vi "Motion Magic.vi"(0 "In":dbl(knob) scale=-360.0..360.0, 1 "Cluster":T1={"kp"=0.28, "ki"=0.0, "kd"=0.02, "kv"=0.104, "ka"=0.0}, 2 "Target":dbl, 3 "Max V":dbl format="%#_13g", 4 "Velocity":dbl format="%#_13g", 5 "Max A":dbl format="%#_13g", 6 "Reset":bool) -> (7 "Output":dbl(knob) scale=-1.0..1.0, 8 "Error":dbl)   [LabVIEW 2017]
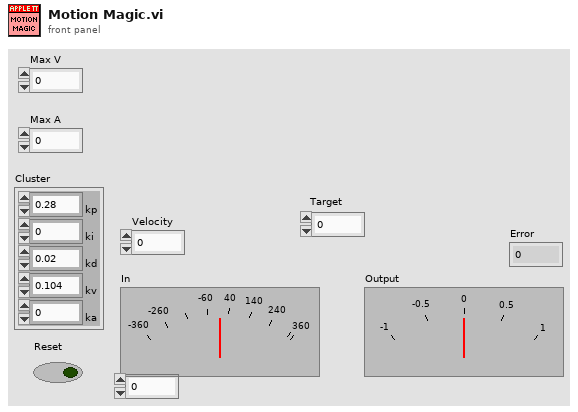
[diagram p1: front panel]
types:
  T1 = cluster{"kp":dbl, "ki":dbl, "kd":dbl, "kv":dbl, "ka":dbl}
  T2 = cluster{"tS":dbl, "tE":dbl, "tC":dbl, "xS":dbl, "xE":dbl, "xC":dbl}
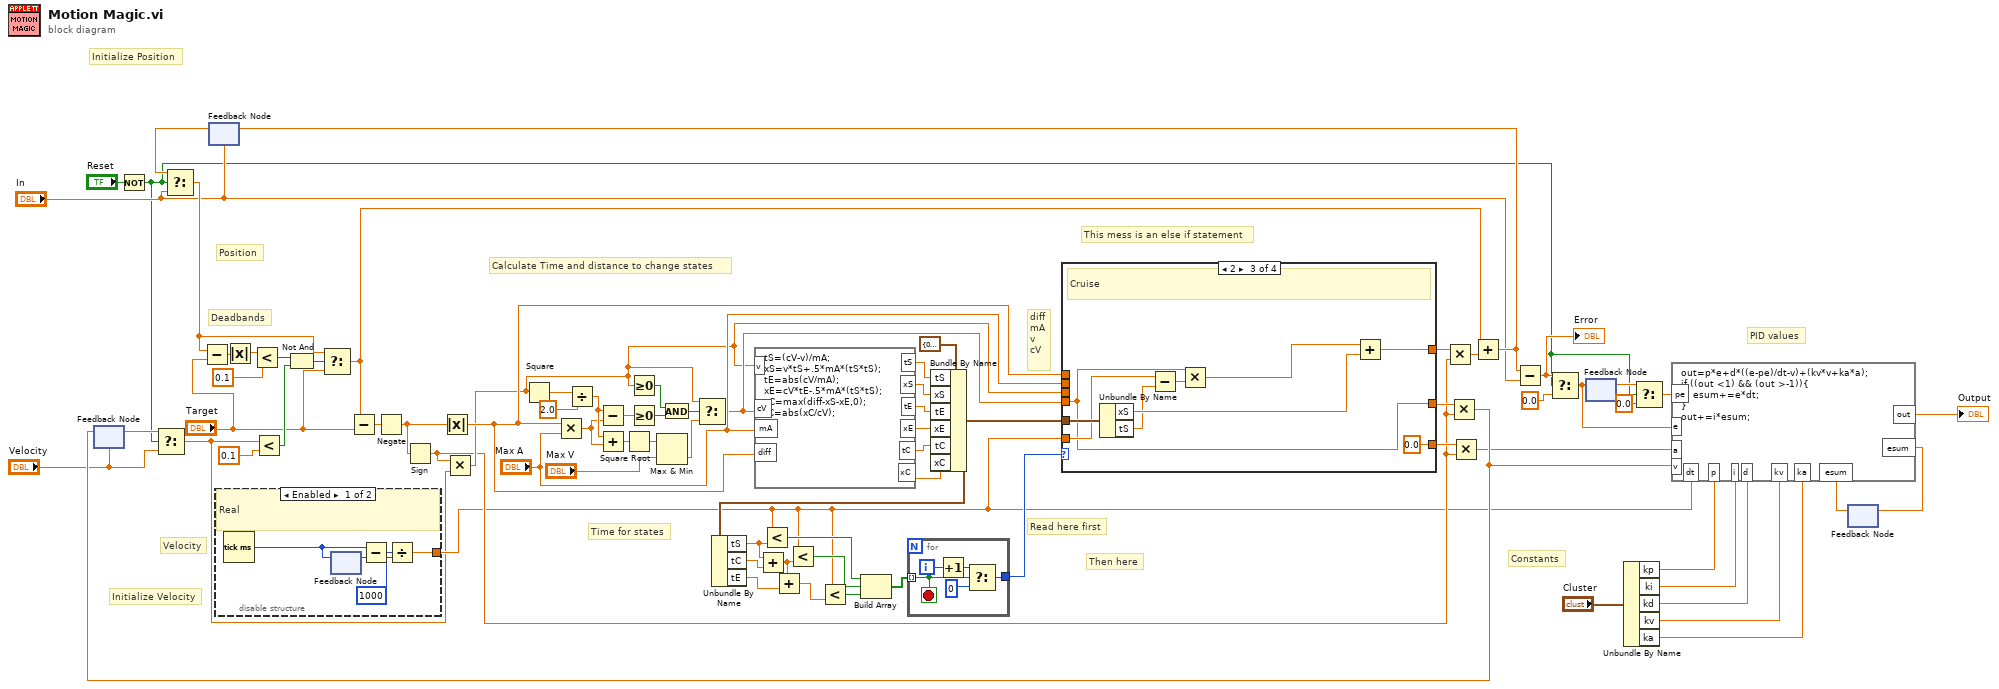
[diagram p0: block diagram]
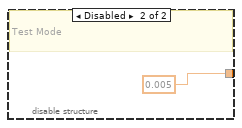
[diagram p2: hidden frame]
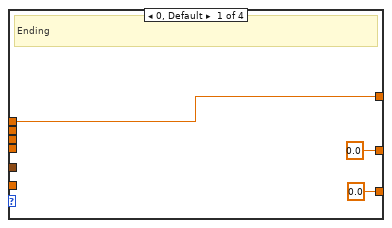
[diagram p3: hidden frame]
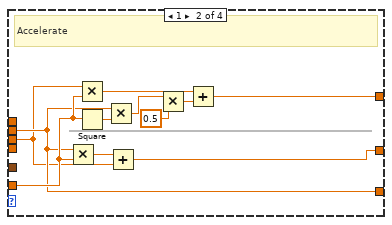
[diagram p4: hidden frame]
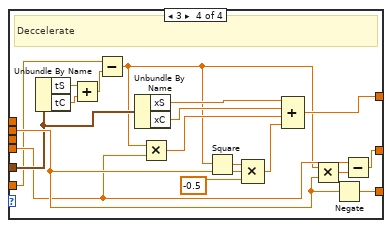
[diagram p5: hidden frame]
diagram:
  # "Time for states"
  # "Constants"
  # "Initialize Position"
  # "Initialize Velocity"
  # "PID values"
  # "Deadbands"
  # "Position"
  # "Velocity"
  # "Calculate Time and distance to change states"
  # "diff\nmA\nv\ncV"
  # "Then here"
  # "Read here first"
  # "This mess is an else if statement"
  n1 = feedback #1("Velocity") -> (w76:dbl)
  n2 = Not(x="Reset") -> (.not. x?=w2:bool)
  n3 = Select(t=w76, s=w2, f="Velocity") -> (s? t:f=w11:dbl)
  n4 = feedback #2("In") -> (w18:dbl)
  n5 = Select(t=w18, s=w2, f="In") -> (s? t:f=w13:dbl)
  n6 = Subtract(x=w13, y="Target") -> (x-y=w34:dbl)
  n7 = disable-structure "Diagram Disable Structure" shown="Enabled" {
    disable-tunnel: [w78 0.005] -> w16
    frame Enabled {
      # "Real"
      n8 = Tick Count (ms)() -> (millisecond timer value=w80:u32)
      n9 = feedback #3() -> (w79:u32)  [unwired: 1 in]
      n10 = feedback-in #3(w80) -> ()
      n11 = Subtract(x=w80, y=w79) -> (x-y=w82:u32)
      n12 = Divide(x=w82, y=1000) -> (x/y=w78:dbl)
    }
    frame Disabled {
      # "Test Mode"
    }
  }
  n13 = Absolute Value(x=w34) -> (abs(x)=w32:dbl)
  n14 = Less?(x=w32, y=0.1) -> (x < y?=w31:bool)
  n15 = Less?(x=w11, y=0.1) -> (x < y?=w29:bool)
  n16 = Not And(1:w29, 2:w31) -> (0:w8:bool)
  n17 = Select(t=w13, s=w8, f="Target") -> (s? t:f=w22:dbl)
  n18 = Subtract(x=w22, y="Target") -> (x-y=w28:dbl)
  n19 = Negate(x=w28) -> (-x=w19:dbl)
  n20 = Sign(1:w19) -> (0:w20:dbl)
  n21 = Absolute Value(x=w19) -> (abs(x)=w46:dbl)
  n22 = Multiply(x=w20, y=w11) -> (x*y=w25:dbl)
  n23 = Square(x=w25) -> (x^2=w75:dbl)
  n24 = Multiply(x=w46, y="Max A") -> (x*y=w67:dbl)
  n25 = Divide(x=w75, y=2.0) -> (x/y=w68:dbl)
  n26 = Subtract(x=w68, y=w67) -> (x-y=w15:dbl)
  n27 = Add(x=w68, y=w67) -> (x+y=w14:dbl)
  n28 = Square Root(x=w14) -> (sqrt(x)=w21:dbl)
  n29 = Greater Or Equal To 0?(x=w25) -> (x >= 0?=w72:bool)
  n30 = Greater Or Equal To 0?(x=w15) -> (x >= 0?=w73:bool)
  n31 = Max & Min(x=w21, y="Max V") -> (min(x,y)=w70:dbl)  [unwired: 1 out]
  n32 = And(x=w72, y=w73) -> (x .and. y?=w71:bool)
  n33 = Select(t=w25, s=w71, f=w70) -> (s? t:f=w49:dbl)
  n34 = formula code="tS=(cV-v)/mA;\nxS=v*tS+.5*mA*(tS*tS);\ntE=abs(cV/mA);\nxE=cV*tE-.5*mA*(tS*tS);\nxC=max(diff-xS-xE,0);\ntC=abs(xC/cV);"("v"=w25, "cV"=w49, "mA"="Max A", "diff"=w46) -> ("tS"=w66:dbl, "xS"=w61:dbl, "tE"=w60:dbl, "xC"=w63:dbl, "xE"=w65:dbl, "tC"=w64:dbl)
  n35 = Bundle By Name(cluster=T2 {"tS"=0.0, "tE"=0.0, "tC"=0.0, "xS"=0.0, "xE"=0.0, "xC"=0.0} ("input cluster"), "tS"=w66, "xS"=w61, "tE"=w60, "xE"=w65, "tC"=w64, "xC"=w63) -> (w48:T2)
  n36 = Unbundle By Name(w48) -> ("tS"=w58:dbl, "tC"=w56:dbl, "tE"=w54:dbl)
  n37 = Add(x=w58, y=w56) -> (x+y=w55:dbl)
  n38 = Less?(x=w16, y=w58) -> (x < y?=w59:bool)
  n39 = Add(x=w55, y=w54) -> (x+y=w52:dbl)
  n40 = Less?(x=w16, y=w55) -> (x < y?=w57:bool)
  n41 = Less?(x=w16, y=w52) -> (x < y?=w53:bool)
  n42 = Build Array(w59, w57, w53) -> (w50:bool[])
  n43 = for {
    tunnel: w50 -> [w84] mode=indexing
    tunnel: [w87] -> w47
    i -> [w88]
    stop <- w84 stop-if-true
    n44 = Increment(x=w88) -> (x+1=w86:i32)
    n45 = Select(t=w86, s=w84, f=0) -> (s? t:f=w87:i32)
  }
  n46 = case shown="2" w47 {
    tunnel: w49 -> [_ _ w105 w118]
    tunnel: w25 -> [_ w92 _ _]
    tunnel: "Max A" -> [_ w93 _ w124]
    tunnel: w48 -> [_ _ w110 w121]
    tunnel: w16 -> [_ w96 w108 w112]
    tunnel: w46 -> [w90 _ _ _]
    tunnel: [0.0 w93 0.0 w129] -> w42
    tunnel: [w90 w94 w103 w122] -> w45
    tunnel: [0.0 w101 w105 w127] -> w43
    frame 0, Default {
      # "Ending"
    }
    frame 1 {
      # "Accelerate"
      n47 = Multiply(x=w93, y=w96) -> (x*y=w102:dbl)
      n48 = Multiply(x=w92, y=w96) -> (x*y=w95:dbl)
      n49 = Square(x=w96) -> (x^2=w100:dbl)
      n50 = Multiply(x=w93, y=w100) -> (x*y=w99:dbl)
      n51 = Add(x=w102, y=w92) -> (x+y=w101:dbl)
      n52 = Multiply(x=w99, y=0.5) -> (x*y=w97:dbl)
      n53 = Add(x=w95, y=w97) -> (x+y=w94:dbl)
    }
    frame 2 {
      # "Cruise"
      n54 = Unbundle By Name(w110) -> ("xS"=w109:dbl, "tS"=w107:dbl)
      n55 = Subtract(x=w108, y=w107) -> (x-y=w106:dbl)
      n56 = Multiply(x=w105, y=w106) -> (x*y=w104:dbl)
      n57 = Add(x=w104, y=w109) -> (x+y=w103:dbl)
    }
    frame 3 {
      # "Deccelerate"
      n58 = Unbundle By Name(w121) -> ("tS"=w116:dbl, "tC"=w115:dbl)
      n59 = Add(x=w116, y=w115) -> (x+y=w114:dbl)
      n60 = Subtract(x=w112, y=w114) -> (x-y=w113:dbl)
      n61 = Unbundle By Name(w121) -> ("xS"=w120:dbl, "xC"=w119:dbl)
      n62 = Multiply(x=w113, y=w118) -> (x*y=w117:dbl)
      n63 = Square(x=w113) -> (x^2=w123:dbl)
      n64 = Compound Arithmetic op=MULTIPLY(w123, w124, -0.5) -> (w126:dbl)
      n65 = Compound Arithmetic op=ADD(w120, w119, w117, w126) -> (w122:dbl)
      n66 = Multiply(x=w113, y=w124) -> (x*y=w128:dbl)
      n67 = Negate(x=w124) -> (-x=w129:dbl)
      n68 = Subtract(x=w118, y=w128) -> (x-y=w127:dbl)
    }
  }
  n69 = Multiply(x=w45, y=w20) -> (x*y=w44:dbl)
  n70 = Multiply(x=w43, y=w20) -> (x*y=w77:dbl)
  n71 = feedback-in #1(w77) -> ()
  n72 = Multiply(x=w42, y=w20) -> (x*y=w41:dbl)
  n73 = Add(x=w22, y=w44) -> (x+y=w17:dbl)
  n74 = feedback-in #2(w17) -> ()
  n75 = Subtract(x=w17, y="In") -> (x-y=w7:dbl)
  "Error" <- w7
  n76 = Select(t=w7, s=w2, f=0.0) -> (s? t:f=w1:dbl)
  n77 = feedback #4() -> (w27:dbl)  [unwired: 1 in]
  n78 = feedback-in #4(w1) -> ()
  n79 = Unbundle By Name("Cluster") -> ("kp"=w40:dbl, "ki"=w39:dbl, "kd"=w38:dbl, "kv"=w37:dbl, "ka"=w36:dbl)
  n80 = Select(t=w27, s=w2, f=0.0) -> (s? t:f=w9:dbl)
  n81 = feedback #5() -> (w35:dbl)  [unwired: 1 in]
  n82 = formula code="out=p*e+d*((e-pe)/dt-v)+(kv*v+ka*a);\nif ((out <1) && (out >-1)){\n    esum+=e*dt;\n}\nout+=i*esum;"("dt"=w16, "e"=w1, "pe"=w9, "v"=w77, "a"=w41, "p"=w40, "i"=w39, "d"=w38, "kv"=w37, "ka"=w36, "esum"=w35) -> ("out"=→"Output":dbl, "esum"=w26:dbl)
  n83 = feedback-in #5(w26) -> ()
